vi "VL53L0X_StaticInit.vi"(11 "REV2mDistanceSensorDevRef":T1) -> (3 "REV2mDistanceSensorDevRef Out":T1)   [LabVIEW 2019, in "DistanceSensorDriver.lvlib"]
uses:
  DistanceSensorDriver.lvlib
  Typedef/REV2mDistanceSensorDevRef.ctl
  Typedef/Ports.ctl
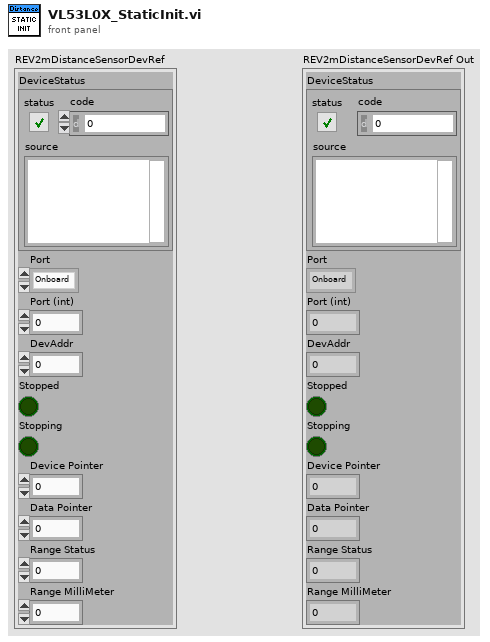
[diagram p1: front panel]
types:
  T1 = typedef "DistanceSensorDriver.lvlib/REV2mDistanceSensorDevRef.ctl" = cluster{"DeviceStatus":errorcluster, "Port":T2, "Port (int)":i32, "DevAddr":i32, "Stopped":bool, "Stopping":bool, "Device Pointer":u64, "Data Pointer":u64, "Range Status":u8, "Range MilliMeter":u16}
  T2 = typedef "DistanceSensorDriver.lvlib/Ports.ctl" = enum32{"Onboard", "MXP"}
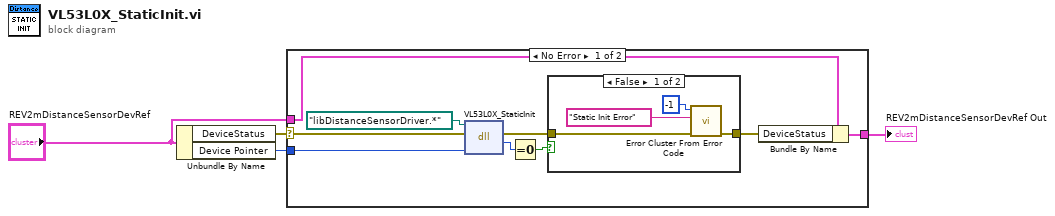
[diagram p0: block diagram]
diagram:
  n1 = Unbundle By Name("REV2mDistanceSensorDevRef") -> ("DeviceStatus"=w1:errorcluster, "Device Pointer"=w4:u64)
  n2 = case shown="No Error" w1 {
    selector: w1 -> [w5 _]
    tunnel: w4 -> [w8 _]
    tunnel: [w7 w19] -> w3
    tunnel: "REV2mDistanceSensorDevRef" -> [w6 w19]
    frame No Error {
      n3 = dll-call lib="?" fn="VL53L0X_StaticInit"(path in=path "libDistanceSensorDriver.*", error in=w5, "Dev"=w8) -> (error out=w9:errorcluster, "Status"=w10:i32)  [unwired: 2 in, 1 out]
      n4 = Equal To 0?(x=w10) -> (x = 0?=w13:bool)
      n5 = case shown="False" w13 {
        tunnel: w9 -> [w14 w18]
        tunnel: [w17 w18] -> w12
        frame False {
          n6 = call <vilib>:"Error Cluster From Error Code.vi"("error in (no error)"=w14, "error message (\"\")"="Static Init Error" ("error message (\"\")"), "error code (0)"=-1) -> ("error out"=w17:errorcluster)  [unwired: 6 in]
        }
        frame True {
        }
      }
      n7 = Bundle By Name(cluster=w6, "DeviceStatus"=w12) -> (w7:T1)
    }
    frame Error {
    }
  }
  "REV2mDistanceSensorDevRef Out" <- w3
